vi "Main.vi"() -> ()   [LabVIEW 2020]
doc: "Cet exemple de projet Mesure continue est basé sur le modèle Gestionnaire de messages dans une file d'attente.\n\nLa boucle de gestion d'événements génère des messages en fonction des actions sur l'interface utilisateur.\n\nLa boucle de gestion de messages traite les messages générés par la boucle de gestion d'événements ou par d'autres messages. Il y a aussi des sous-VIs de boucle de gestion de messages d'acquisition et d'enregistrement, ainsi qu'une boucle de mise à jour du graphe déroulant."
uses:
  Settings/Settings.ctl
  Acquisition/Hardware Configuration.ctl
  Acquisition/Signal Type.ctl
  Logging/Logging Configuration.ctl
  controls/UI Data.ctl
  controls/UI State.ctl
  support/Message Queue/Enqueue Message (Single).vi
  support/Message Queue/Enqueue Message (Array).vi
  <vilib>/Utility/error.llb/Error Cluster From Error Code.vi
  <vilib>/ErrorRing/Error Ring.xnode
  Acquisition/Acquisition.lvlib
  Logging/Logging.lvlib
  Settings/Settings.lvlib
  support/User Event - Stop/User Event - Stop.lvlib
  support/Message Queue/Message Queue.lvlib
  Settings/Settings Dialog.vi
panel:
  in  "Panneaux":T1(tab)
  out "Chaîne":string
  in  "Moyennage sélectionneur":bool
  in  "Choix moyennage":dbl
  in  "Mode longueur d'onde":bool=TRUE
  in  "Sélectionneur de longueur d'onde":dbl=500.0 min=500.0 max=2500.0 step=1.0
  in  "Longueur d'onde":bool
  out "Données":waveform(dbl)[](graph)
  out "État":string
  in  "Quitter":bool
  in  "Arrêter":bool
  in  "Démarrer":bool
  in  "Paramètres":bool
  out "Tableau 2":dbl[](array[numeric])
  # "MAPA Tech"
  # "Automatique"
  # "Manuel"
  # "MAPA Tech"
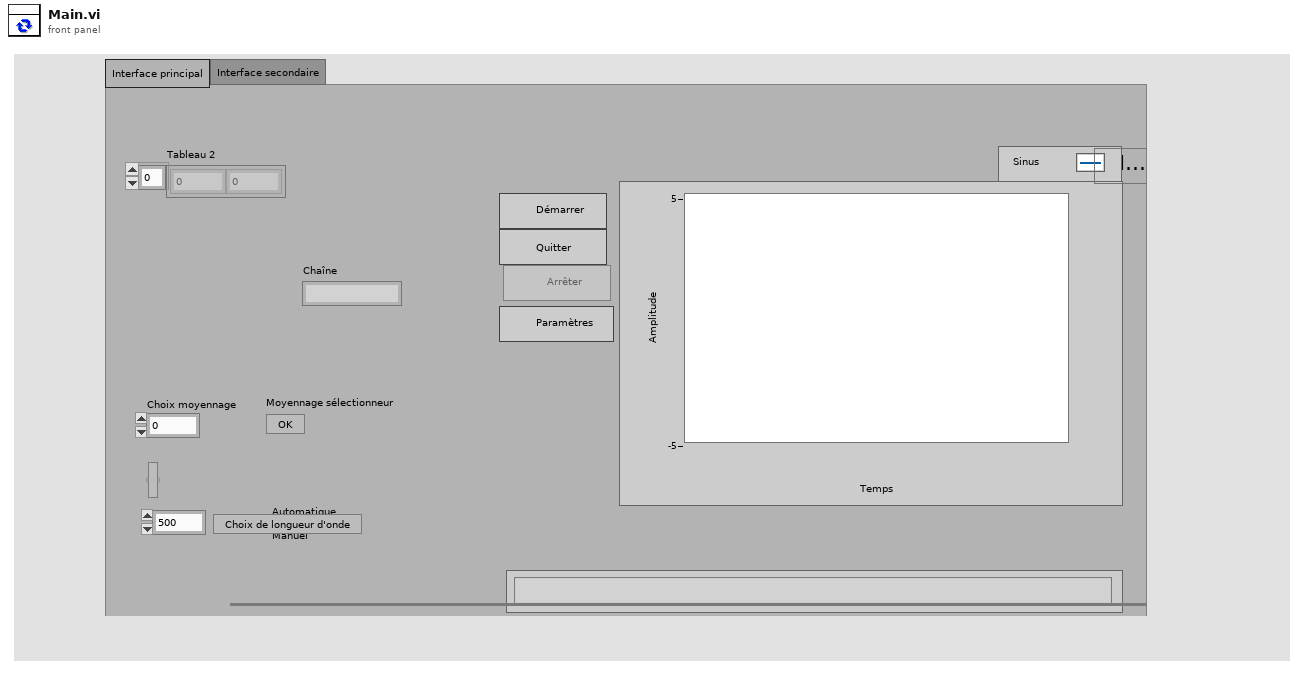
[diagram p1: front panel]
types:
  T1 = enum32{"Interface principal", "Interface secondaire"}
  T2 = typedef "UI State.ctl" = enum16{"Idle", "Acquiring and Logging", "Waiting for Exit", "Waiting for Exit (Acq Stopped)", "Waiting for Exit (Log Stopped)", "Waiting for Stop", "Waiting for Stop (Acq Stopped)", "Waiting for Stop (Log Stopped)"}
  T3 = typedef "UI Data.ctl" = cluster{"Réf. de Démarrer":refnum<vi>, "Réf. d'Arrêter":refnum<vi>, "Réf. de Paramètres":refnum<vi>, "Réf. de Quitter":refnum<vi>, "Réf. d'état":refnum<vi>, "Réf. de données":refnum<vi>, "Ref. longueur d'onde":refnum<vi>, "Ref. Choix mode longueur d'onde":refnum<vi>, "Ref. Moyennage sélectionneur":refnum<vi>}
  T4 = typedef "Settings.lvlib/Settings.ctl" = cluster{"Configuration du matériel":T5, "Configuration de l'enregistrement":T7, "Cluster test":cluster{"Numérique":dbl, "Numérique 2":dbl}, "Mode de longueur d'onde":cluster{"Choix du mode":bool}}
  T5 = typedef "Acquisition.lvlib/Hardware Configuration.ctl" = cluster{"Refnum de matériel <À remplacer>":string, "Type de signal <À remplacer>":T6}
  T6 = typedef "Acquisition.lvlib/Signal Type.ctl" = enum16{"Sine Wave", "Square with Noise", "Signal triangulaire", "Simulation DAQ"}
  T7 = typedef "Logging.lvlib/Logging Configuration.ctl" = cluster{"Chemin de base du fichier journal":path, "Référence de fichier TDMS":refnum<k34>}
  T8 = cluster{"état":bool, "code":i32, "source":string}
  T9 = typedef "Message Queue.lvlib/All Message Queues.ctl" = cluster{"IU":refnum<queue>, "Acquisition":refnum<queue>, "Enregistrement":refnum<queue>}
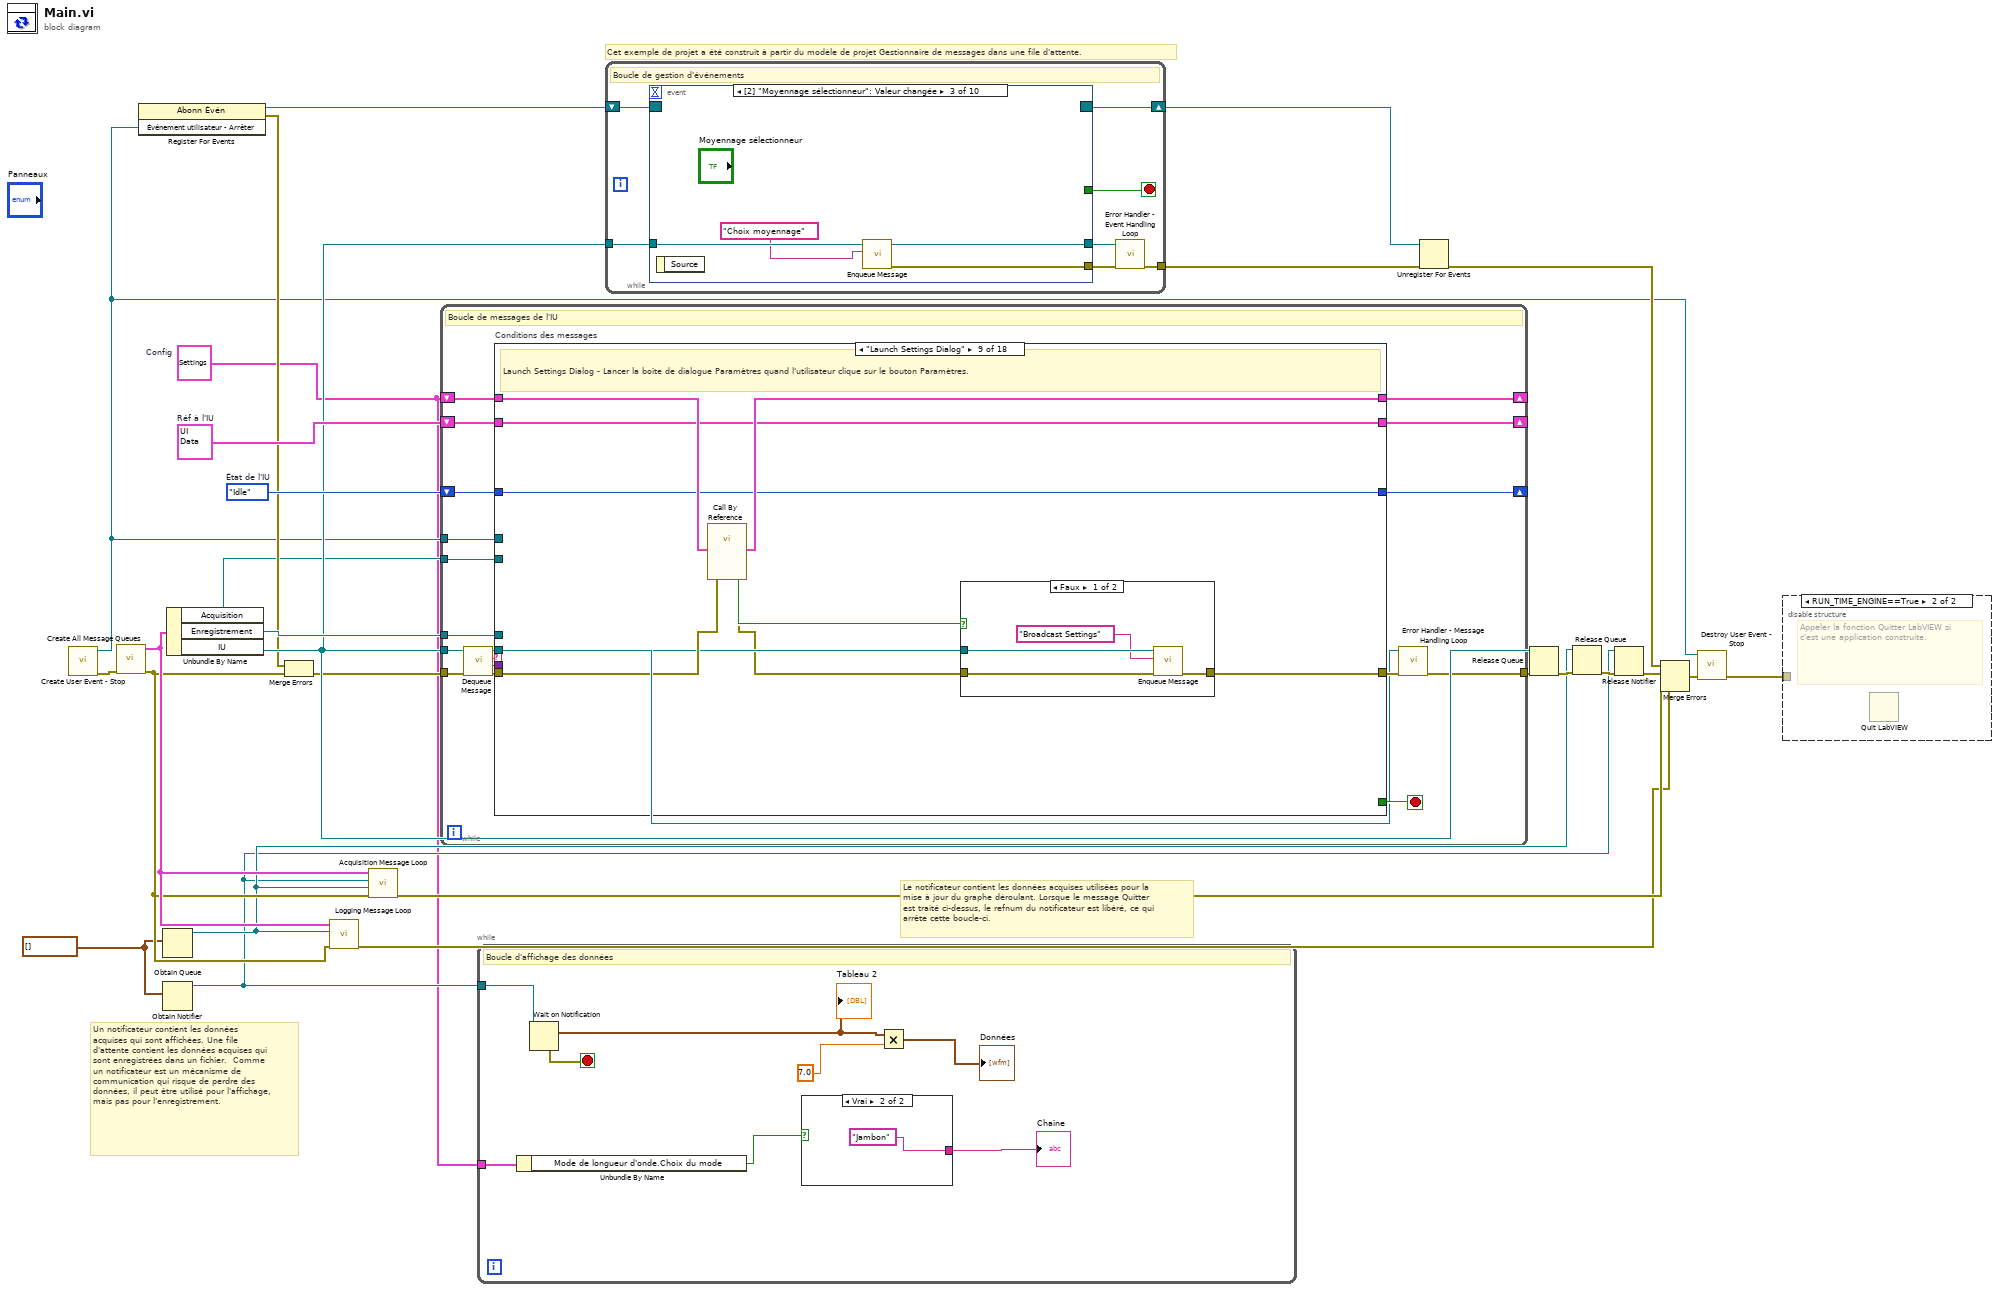
[diagram p0: block diagram]
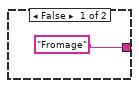
[diagram p3: hidden frame]
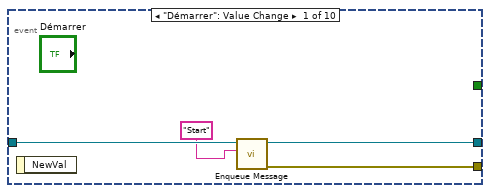
[diagram p4: hidden frame]
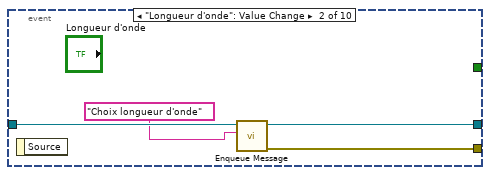
[diagram p5: hidden frame]
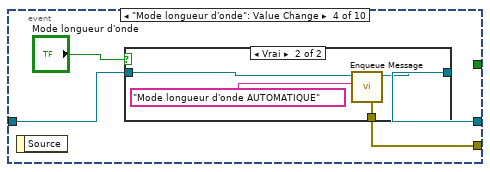
[diagram p6: hidden frame]
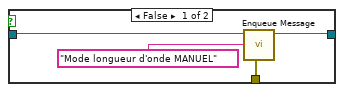
[diagram p7: hidden frame]
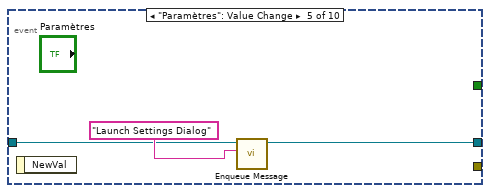
[diagram p8: hidden frame]
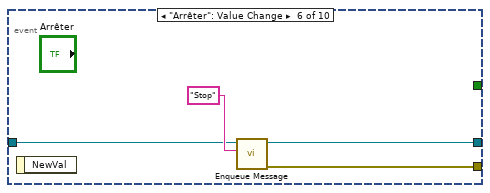
[diagram p9: hidden frame]
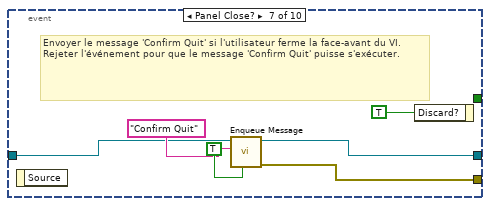
[diagram p10: hidden frame]
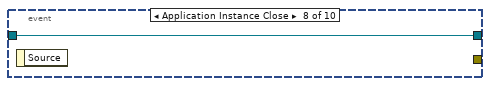
[diagram p11: hidden frame]
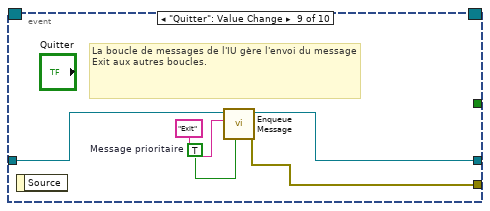
[diagram p12: hidden frame]
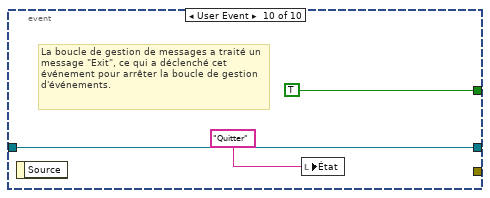
[diagram p13: hidden frame]
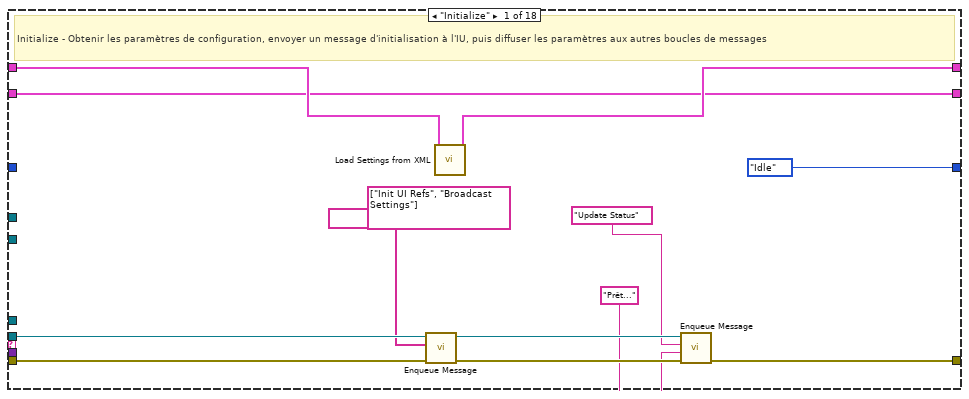
[diagram p14: hidden frame]
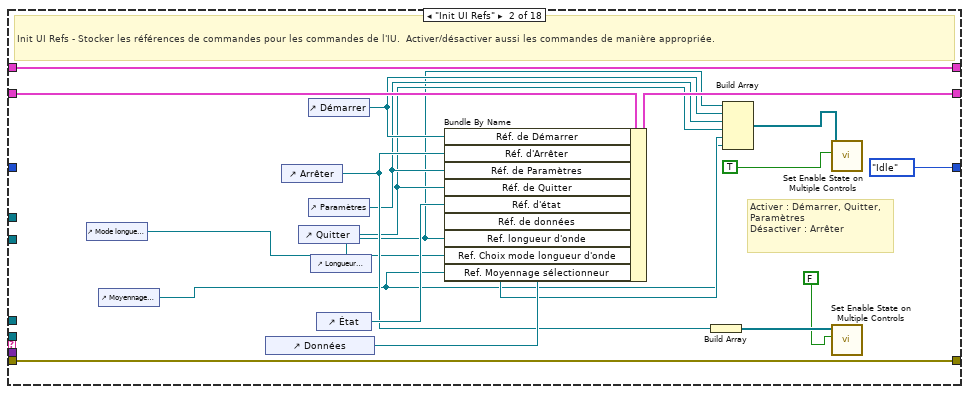
[diagram p15: hidden frame]
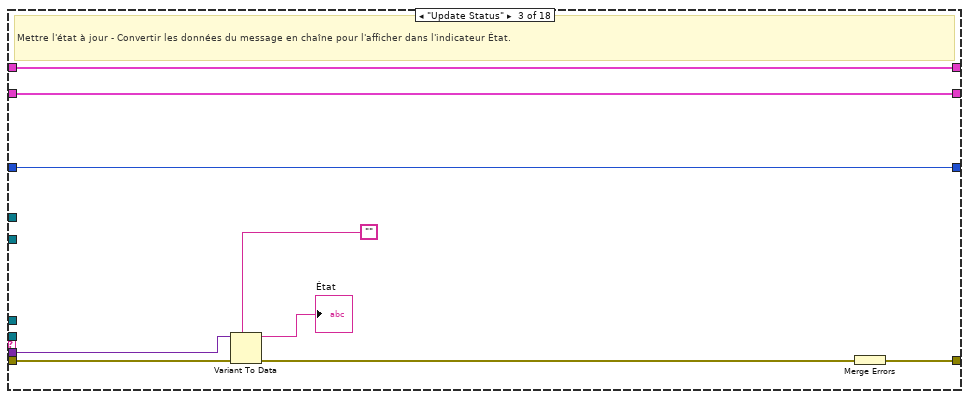
[diagram p16: hidden frame]
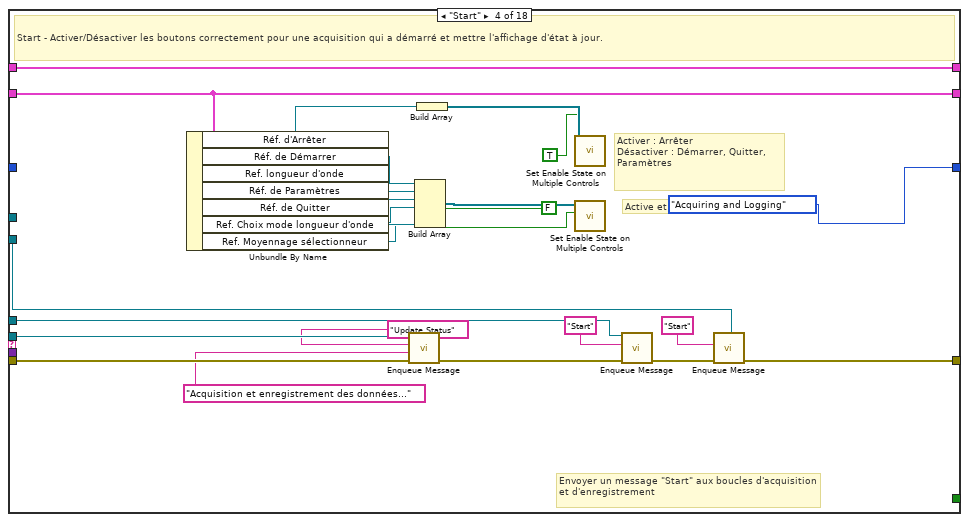
[diagram p17: hidden frame]
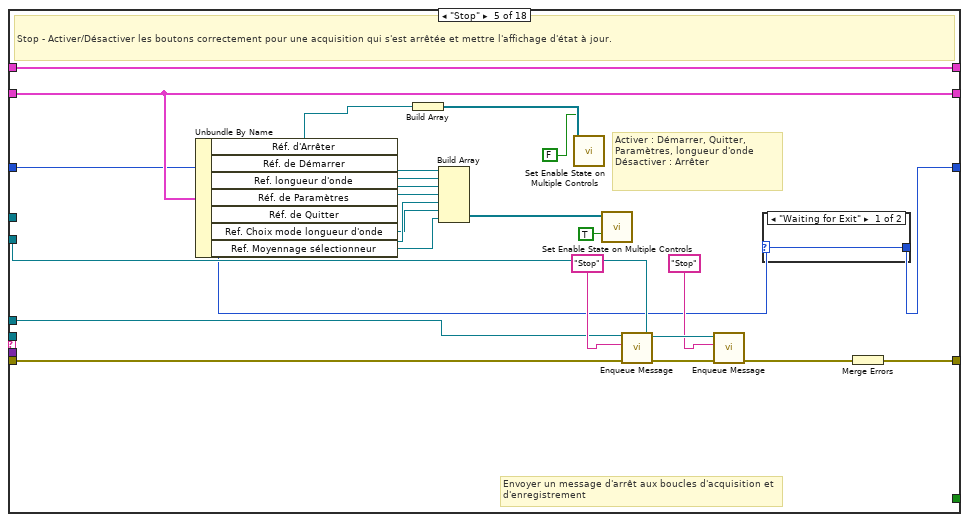
[diagram p18: hidden frame]
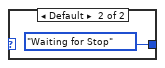
[diagram p19: hidden frame]
diagram:
  w16 = UI_State."Idle"  # État de l'IU
  w2 = waveform(dbl)[] []
  w18 = T3 {"Réf. de Démarrer"=refnum, "Réf. d'Arrêter"=refnum, "Réf. de Paramètres"=refnum, "Réf. de Quitter"=refnum, "Réf. d'état"=refnum, "Réf. de données"=refnum, "Ref. longueur d'onde"=refnum, "Ref. Choix mode longueur d'onde"=refnum, "Ref. Moyennage sélectionneur"=refnum}  # Réf à l'IU
  w1 = T4 {"Configuration du matériel"={"Refnum de matériel <À remplacer>"="", "Type de signal <À remplacer>"=enum."Simulation DAQ"}, "Configuration de l'enregistrement"={"Chemin de base du fichier journal"=path "", "Référence de fichier TDMS"=refnum}, "Cluster test"={"Numérique"=15.0, "Numérique 2"=0.0}, "Mode de longueur d'onde"={"Choix du mode"=TRUE}}  # Config
  # "Cet exemple de projet a été construit à partir du modèle de projet Gestionnaire de messages dans une file d'attente."
  # "Un notificateur contient les données acquises qui sont affichées. Une file d'attente contient les données acquises qui sont enregistrées dans un fichier.  Comme un notificateur est un mécanisme de communication qui risque de perdre des données, il peut être utilisé pour l'affichage, mais pas pour l'enregistrement."
  # "Le notificateur contient les données acquises utilisées pour la mise à jour du graphe déroulant. Lorsque le message Quitter est traité ci-dessus, le refnum du notificateur est libéré, ce qui arrête cette boucle-ci."
  n1 = call "Create User Event - Stop.vi"() -> ("error out"=w24:T8, "Événement utilisateur - Arrêter"=w3:refnum<user-event>)  [unwired: 10 in]
  n2 = call "Create All Message Queues.vi"("error in (no error)"=w24) -> ("error out"=w21:T8, "Files d'attente de messages en sortie"=w23:T9)  [unwired: 9 in]
  n3 = register-events(w3) -> (reference out=w7:refnum<event-registration>, error out=w5:errorcluster)  [unwired: 2 in]
  n4 = Obtain Queue(element data type=w2) -> (queue out=w9:refnum<queue>)  [unwired: 4 in, 2 out]
  n5 = Obtain Notifier(notification data type=w2) -> (notifier out=w8:refnum<notifier>)  [unwired: 3 in, 2 out]
  n6 = Unbundle By Name(w23) -> ("Acquisition"=w4:refnum<queue>, "Enregistrement"=w17:refnum<queue>, "IU"=w14:refnum<queue>)
  n7 = Merge Errors(w5, w21) -> (w6:errorcluster)
  n8 = call "Logging Message Loop.vi"("error in (no error)"=w21, "File d'attente de données"=w9, "Files d'attente de messages"=w23) -> ("error out"=w22:T8)  [unwired: 8 in]
  n9 = call "Acquisition Message Loop.vi"("error in (no error)"=w21, "File d'attente de données"=w9, "Notificateur de données"=w8, "Files d'attente de messages"=w23) -> ("error out"=w25:T8)  [unwired: 7 in]
  n10 = while {
    tunnel: w14 -> [w39]
    tunnel: w3 -> [w44]
    shift-right: [w38] -> _
    shift-left: w1 -> [w37]
    shift-right: [w35] -> _
    shift-left: w18 -> [w36]
    tunnel: w4 -> [w34]
    tunnel: w17 -> [w33]
    shift-right: [w28] -> _
    shift-left: w16 -> [w29]
    tunnel: w6 -> [w43]
    tunnel: [w32] -> w27
    stop <- w45 stop-if-true
    # "Boucle de messages de l'IU"
    n11 = call "Dequeue Message.vi"("error in (no error)"=w43, "File d'attente de messages"=w39) -> ("error out"=w42:T8, "Données de message"=w40:variant, "Message"=w41:string, "File d'attente de message dup."=w30:refnum<queue>)  [unwired: 6 in]
    n12 = case "Conditions des messages" shown="\"Launch Settings Dialog\"" w41 {
      selector: w41 -> [_ _ _ _ _ _ _ _ _ _ _ _ _ _ _ _ _ w347]
      tunnel: w30 -> [w49 _ _ w109 _ w137 w162 _ w204 _ w225 _ _ w288 w308 w325 w342 _]
      tunnel: w42 -> [w48 w75 w83 w108 w131 w138 w163 w192 w206 w213 w224 w253 w270 w291 w311 w328 w345 _]
      tunnel: [w53 w75 w84 w93 w132 w135 w160 w198 w199 w216 w223 w263 w269 w290 w310 w327 w344 w346] -> w31
      tunnel: [_ _ _ _ _ _ _ _ _ _ _ TRUE _ _ _ _ _ _] -> w45
      tunnel: w40 -> [_ _ w82 _ _ _ _ _ _ w217 _ w251 _ _ _ _ _ _]
      tunnel: w44 -> [_ _ _ _ _ _ _ _ _ _ _ w264 _ _ _ _ _ _]
      tunnel: [w56 w74 w78 w107 w130 w141 w166 w196 w203 w221 w228 w262 w268 w289 w309 w326 w343 w350] -> w38
      tunnel: w37 -> [w57 w74 w78 w107 w130 w141 w166 w196 w207 w221 w228 w262 w268 w289 w309 w326 w343 w350]
      tunnel: w36 -> [w50 w73 w77 w104 w129 w140 w165 w191 w201 w220 w227 w261 w267 w279 w300 w319 w336 w349]
      tunnel: [w50 w70 w77 w104 w129 w140 w165 w191 w201 w220 w227 w261 w267 w279 w300 w319 w336 w349] -> w35
      tunnel: w34 -> [_ _ _ w92 w118 _ _ w190 _ _ _ w260 _ _ _ _ _ _]
      tunnel: w33 -> [_ _ _ w95 w121 _ _ w185 _ _ _ w259 _ _ _ _ _ _]
      tunnel: w29 -> [_ _ w76 _ w115 w139 w164 w189 w200 w215 w226 _ w266 _ _ _ _ w348]
      tunnel: [UI_State."Idle" ("UI State") UI_State."Idle" ("UI State") w76 UI_State."Acquiring and Logging" ("UI State") w116 w136 w161 w189 w200 w215 w222 UI_State."Idle" ("UI State") w266 UI_State."Acquiring and Logging" ("UI State") UI_State."Acquiring and Logging" ("UI State") UI_State."Acquiring and Logging" ("UI State") UI_State."Acquiring and Logging" ("UI State") w348] -> w28
      frame "Initialize" {
        # "Initialize - Obtenir les paramètres de configuration, envoyer un message d'initialisation à l'IU, puis diffuser les paramètres aux autres boucles de messages"
        n13 = call-poly "Enqueue Message.vi"("error in (no error)"=w48, "Tableau de messages"=string[] ["Init UI Refs", "Broadcast Settings"], "File d'attente de messages"=w49) -> ("error out"=w55:T8, "File d'attente de message dup."=w54:refnum<queue>)  [unwired: 7 in]
        n14 = call "Load Settings from XML.vi"("Paramètres en entrée"=w57) -> ("Paramètres en sortie"=w56:T4)  [unwired: 9 in, 1 out]
        n15 = call-poly "Enqueue Message.vi"("error in (no error)"=w55, "Données de message"="Prêt..." ("Ready..."), "Message"="Update Status", "File d'attente de messages"=w54) -> ("error out"=w53:T8)  [unwired: 6 in, 1 out]
      }
      frame "Init UI Refs" {
        # "Activer : Démarrer, Quitter, Paramètres\nDésactiver : Arrêter"
        # "Init UI Refs - Stocker les références de commandes pour les commandes de l'IU.  Activer/désactiver aussi les commandes de manière appropriée."
        n16 = control-ref of="Mode longueur d'onde"() -> (w59:refnum<vi>)
        n17 = control-ref of="Moyennage sélectionneur"() -> (w58:refnum<vi>)
        n18 = control-ref of="Données"() -> (w71:refnum<vi>)
        n19 = control-ref of="Arrêter"() -> (w65:refnum<vi>)
        n20 = control-ref of="Quitter"() -> (w62:refnum<vi>)
        n21 = control-ref of="Démarrer"() -> (w64:refnum<vi>)
        n22 = control-ref of="Paramètres"() -> (w63:refnum<vi>)
        n23 = control-ref of="Longueur d'onde"() -> (w60:refnum<vi>)
        n24 = control-ref of="État"() -> (w72:refnum<vi>)
        n25 = Bundle By Name(cluster=w73, "Réf. de Démarrer"=w64, "Réf. d'Arrêter"=w65, "Réf. de Paramètres"=w63, "Réf. de Quitter"=w62, "Réf. d'état"=w72, "Réf. de données"=w71, "Ref. longueur d'onde"=w60, "Ref. Choix mode longueur d'onde"=w59, "Ref. Moyennage sélectionneur"=w58) -> (w70:T3)
        n26 = Build Array(w65) -> (w67:refnum<vi>[])
        n27 = Build Array(w60, w64, w63, w62, w59, w58) -> (w68:refnum<vi>[])
        n28 = call "Set Enable State on Multiple Controls.vi"("Activé ?"=TRUE ("Enable?"), "Commandes"=w68) -> ()  [unwired: 10 in]
        n29 = call "Set Enable State on Multiple Controls.vi"("Activé ?"=FALSE ("Enable?"), "Commandes"=w67) -> ()  [unwired: 10 in]
      }
      frame "Update Status" {
        # "Mettre l'état à jour - Convertir les données du message en chaîne pour l'afficher dans l'indicateur État."
        n30 = Variant To Data(error in=w83, type="" ("Empty String Constant"), Variant=w82) -> (data=→"État":string, error out=w80:errorcluster)
        n31 = Merge Errors(w80) -> (w84:errorcluster)
      }
      frame "Start" {
        # "Active et désactive les boutons!"
        # "Envoyer un message \"Start\" aux boucles d'acquisition et d'enregistrement"
        # "Activer : Arrêter\nDésactiver : Démarrer, Quitter, Paramètres"
        # "Start - Activer/Désactiver les boutons correctement pour une acquisition qui a démarré et mettre l'affichage d'état à jour."
        n32 = Unbundle By Name(w104) -> ("Réf. d'Arrêter"=w99:refnum<vi>, "Réf. de Démarrer"=w98:refnum<vi>, "Ref. longueur d'onde"=w89:refnum<vi>, "Réf. de Paramètres"=w88:refnum<vi>, "Réf. de Quitter"=w87:refnum<vi>, "Ref. Choix mode longueur d'onde"=w86:refnum<vi>, "Ref. Moyennage sélectionneur"=w85:refnum<vi>)
        n33 = call-poly "Enqueue Message.vi"("error in (no error)"=w108, "Données de message"="Acquisition et enregistrement des données..." ("Acquiring and Logging..."), "Message"="Update Status", "File d'attente de messages"=w109) -> ("error out"=w97:T8)  [unwired: 6 in, 1 out]
        n34 = Build Array(w98, w89, w88, w87, w86, w85) -> (w102:refnum<vi>[])
        n35 = Build Array(w99) -> (w101:refnum<vi>[])
        n36 = call "Set Enable State on Multiple Controls.vi"("Activé ?"=TRUE ("Enable?"), "Commandes"=w101) -> ()  [unwired: 10 in]
        n37 = call "Set Enable State on Multiple Controls.vi"("Activé ?"=FALSE ("Enable?"), "Commandes"=w102) -> ()  [unwired: 10 in]
        n38 = call-poly "Enqueue Message.vi"("error in (no error)"=w97, "Message"="Start", "File d'attente de messages"=w95) -> ("error out"=w94:T8)  [unwired: 7 in, 1 out]
        n39 = call-poly "Enqueue Message.vi"("error in (no error)"=w94, "Message"="Start", "File d'attente de messages"=w92) -> ("error out"=w93:T8)  [unwired: 7 in, 1 out]
      }
      frame "Stop" {
        # "Envoyer un message d'arrêt aux boucles d'acquisition et d'enregistrement"
        # "Activer : Démarrer, Quitter, Paramètres, longueur d'onde\nDésactiver : Arrêter"
        # "Stop - Activer/Désactiver les boutons correctement pour une acquisition qui s'est arrêtée et mettre l'affichage d'état à jour."
        n40 = Unbundle By Name(w129) -> ("Réf. d'Arrêter"=w124:refnum<vi>, "Réf. de Démarrer"=w123:refnum<vi>, "Ref. longueur d'onde"=w114:refnum<vi>, "Réf. de Paramètres"=w113:refnum<vi>, "Réf. de Quitter"=w112:refnum<vi>, "Ref. Choix mode longueur d'onde"=w111:refnum<vi>, "Ref. Moyennage sélectionneur"=w110:refnum<vi>)
        n41 = Build Array(w124) -> (w126:refnum<vi>[])
        n42 = Build Array(w114, w123, w114, w113, w112, w111, w110) -> (w127:refnum<vi>[])
        n43 = call "Set Enable State on Multiple Controls.vi"("Activé ?"=FALSE ("Enable?"), "Commandes"=w126) -> ()  [unwired: 10 in]
        n44 = call "Set Enable State on Multiple Controls.vi"("Activé ?"=TRUE ("Enable?"), "Commandes"=w127) -> ()  [unwired: 10 in]
        n45 = call-poly "Enqueue Message.vi"("error in (no error)"=w131, "Message"="Stop", "File d'attente de messages"=w121) -> ("error out"=w120:T8)  [unwired: 7 in, 1 out]
        n46 = call-poly "Enqueue Message.vi"("error in (no error)"=w120, "Message"="Stop", "File d'attente de messages"=w118) -> ("error out"=w119:T8)  [unwired: 7 in, 1 out]
        n47 = case shown="\"Waiting for Exit\"" w115 {
          selector: w115 -> [w133 _]
          tunnel: [w133 UI_State."Waiting for Stop" ("UI State")] -> w116
          frame "Waiting for Exit" {
          }
          frame Default {
          }
        }
        n48 = Merge Errors(w119) -> (w132:errorcluster)
      }
      frame "Acquisition Stopped" {
        # "Logique déterminant quelle action entreprendre quand l'acquisition s'est arrêtée."
        n49 = case shown="Par défaut" w139 {
          selector: w139 -> [w143 _ _ _ _]
          tunnel: w138 -> [w142 w145 w147 w153 w159]
          tunnel: w137 -> [_ _ _ w151 w156]
          tunnel: [w143 UI_State."Waiting for Exit (Acq Stopped)" ("UI State") UI_State."Waiting for Stop (Acq Stopped)" ("UI State") UI_State."Idle" ("UI State") UI_State."Idle" ("UI State")] -> w136
          tunnel: [w142 w145 w147 w152 w157] -> w135
          frame Default {
          }
          frame "Waiting for Exit", "Waiting for Exit (Acq Stopped)" {
          }
          frame "Waiting for Stop", "Waiting for Stop (Acq Stopped)" {
          }
          frame "Waiting for Exit (Log Stopped)" {
            # "Si nous attendons pour quitter et que l'enregistrement s'est déjà arrêté, le message \"Acquisition Stopped\" indique qu'il est temps de quitter."
            n50 = call-poly "Enqueue Message.vi"("Message prioritaire ? (F)"=TRUE ("Priority Message? (F)"), "error in (no error)"=w153, "Message"="Exit", "File d'attente de messages"=w151) -> ("error out"=w152:T8)  [unwired: 6 in, 1 out]
          }
          frame "Waiting for Stop (Log Stopped)" {
            # "Si nous attendons pour arrêter et que l'enregistrement s'est déjà arrêté, le message \"Acquisition Stopped\" indique qu'il est temps d'arrêter."
            n51 = call-poly "Enqueue Message.vi"("error in (no error)"=w159, "Données de message"="Prêt..." ("Ready..."), "Message"="Update Status", "File d'attente de messages"=w156) -> ("error out"=w157:T8)  [unwired: 6 in, 1 out]
          }
        }
      }
      frame "Logging Stopped" {
        # "Logique déterminant quelle action entreprendre quand l'enregistrement s'est arrêté."
        n52 = case shown="\"Waiting for Stop (Acq Stopped)\"" w164 {
          selector: w164 -> [w168 _ _ _ _]
          tunnel: w163 -> [w167 w170 w172 w178 w181]
          tunnel: w162 -> [_ _ _ w176 w180]
          tunnel: [w168 UI_State."Waiting for Exit (Log Stopped)" ("UI State") UI_State."Waiting for Stop (Log Stopped)" ("UI State") UI_State."Idle" ("UI State") UI_State."Idle" ("UI State")] -> w161
          tunnel: [w167 w170 w172 w177 w179] -> w160
          frame Default {
          }
          frame "Waiting for Exit", "Waiting for Exit (Log Stopped)" {
          }
          frame "Waiting for Stop", "Waiting for Stop (Log Stopped)" {
          }
          frame "Waiting for Exit (Acq Stopped)" {
            # "Si nous attendons pour quitter et que l'acquisition s'est déjà arrêtée, le message \"Logging Stopped\" indique qu'il est temps de quitter."
            n53 = call-poly "Enqueue Message.vi"("Message prioritaire ? (F)"=TRUE ("Priority Message? (F)"), "error in (no error)"=w178, "Message"="Exit", "File d'attente de messages"=w176) -> ("error out"=w177:T8)  [unwired: 6 in, 1 out]
          }
          frame "Waiting for Stop (Acq Stopped)" {
            # "Si nous attendons pour arrêter et que l'acquisition s'est déjà arrêtée, le message \"Logging Stopped\" indique qu'il est temps d'arrêter."
            n54 = call-poly "Enqueue Message.vi"("error in (no error)"=w181, "Données de message"="Prêt..." ("Ready..."), "Message"="Update Status", "File d'attente de messages"=w180) -> ("error out"=w179:T8)  [unwired: 6 in, 1 out]
          }
        }
      }
      frame "Broadcast settings" {
        w186 = "Update Settings" ("Message")
        # "Broadcast settings - Envoyer le message 'Update Settings' aux boucles de messages d'enregistrement et d'acquisition."
        n55 = Unbundle By Name(w196) -> ("Configuration du matériel"=w195:T5, "Configuration de l'enregistrement"=w194:T7, "Mode de longueur d'onde"=w188:cluster{"Choix du mode":bool})
        n56 = call-poly "Enqueue Message.vi"("Données de message"=w188, "Message"=w186, "File d'attente de messages"=w185) -> ("error out"=w187:T8)  [unwired: 7 in, 1 out]
        n57 = call-poly "Enqueue Message.vi"("Données de message"=w195, "Message"=w186, "File d'attente de messages"=w190) -> ("error out"=w197:T8)  [unwired: 7 in, 1 out]
        n58 = call-poly "Enqueue Message.vi"("error in (no error)"=w197, "Données de message"=w194, "Message"=w186, "File d'attente de messages"=w185) -> ("error out"=w193:T8)  [unwired: 6 in, 1 out]
        n59 = Merge Errors(w187, w193, w192) -> (w198:errorcluster)
      }
      frame "Launch Settings Dialog" {
        # "Launch Settings Dialog - Lancer la boîte de dialogue Paramètres quand l'utilisateur clique sur le bouton Paramètres."
        n60 = call-by-ref "?"("error in (no error)"=w206, "Paramètres en entrée"=w207) -> ("error out"=w202:T8, "Annulation ?"=w205:bool, "Paramètres en sortie"=w203:T4)  [unwired: 8 in, 3 out]
        n61 = case shown="Faux" w205 {
          tunnel: w204 -> [w211 _]
          tunnel: w202 -> [w210 w212]
          tunnel: [w209 w212] -> w199
          frame False {
            n62 = call-poly "Enqueue Message.vi"("error in (no error)"=w210, "Message"="Broadcast Settings", "File d'attente de messages"=w211) -> ("error out"=w209:T8)  [unwired: 7 in, 1 out]
          }
          frame True {
          }
        }
      }
      frame "Error" {
        # "Error - Afficher une boîte de dialogue d'erreur. Ce message est envoyé par les VIs \"Error Handler\" à la fin de l'exécution de chaque boucle de cette application."
        n63 = Variant To Data(error in=w213, type=errorcluster {"status"=FALSE, "code"=0, "source"=""} ("error constant"), Variant=w217) -> (data=w214:errorcluster, error out=w218:errorcluster)
        n64 = call <vilib>:"Simple Error Handler.vi"("error in (no error)"=w214) -> ()  [unwired: 4 in, 5 out]
        n65 = Merge Errors(w218) -> (w216:errorcluster)
      }
      frame "Confirm Quit" {
        # "Confirm Quit - Message qui confirme si l'utilisateur voulait vraiment quitter l'application."
        n66 = case shown="\"Acquiring and Logging\"" w226 {
          tunnel: w225 -> [w234 w238]
          tunnel: w224 -> [w233 w237]
          tunnel: [w232 w236] -> w223
          tunnel: [UI_State."Idle" ("UI State") w235] -> w222
          frame Default {
            # "Si 'Confirm Quit' survient alors que le système est inactif, le message de confirmation est inutile."
            n67 = call-poly "Enqueue Message.vi"("Message prioritaire ? (F)"=TRUE ("Priority Message? (F)"), "error in (no error)"=w233, "Message"="Exit", "File d'attente de messages"=w234) -> ("error out"=w232:T8)  [unwired: 6 in, 1 out]
          }
          frame "Acquiring and Logging" {
            n68 = Two Button Dialog(message="Voulez-vous vraiment quitter en cours d'acquisition ?" ("Confirm Quit Message"), 1:"Non" ("No"), 2:"Oui" ("Yes")) -> (T button?=w239:bool)
            n69 = case shown="Vrai" w239 {
              tunnel: w238 -> [_ w248]
              tunnel: w237 -> [w244 w249]
              tunnel: [w244 w247] -> w236
              tunnel: [UI_State."Acquiring and Logging" ("UI State") UI_State."Waiting for Exit" ("UI State")] -> w235
              frame False {
                # "L'utilisateur ne voulait pas quitter."
              }
              frame True {
                n70 = call-poly "Enqueue Message.vi"("error in (no error)"=w249, "Message"="Stop", "File d'attente de messages"=w248) -> ("error out"=w247:T8)  [unwired: 7 in, 1 out]
              }
            }
          }
        }
      }
      frame "Exit" {
        w255 = TRUE ("Priority Message? (F)")
        w256 = "Exit" ("Message")
        # "Afficher une boîte de dialogue d'erreur si 'Exit' a été appelé suite à une erreur."
        # "Arrêter le VI"
        # "Exit - Envoyer des messages Exit aux boucles d'acquisition et d'enregistrerment, et déclencher l'événement utilisateur pour arrêter la boucle de gestion d'événements."
        n71 = Variant To Data(type=errorcluster {"status"=FALSE, "code"=0, "source"=""} ("error constant"), Variant=w251) -> (data=w250:errorcluster)  [unwired: 1 in, 1 out]
        n72 = call <vilib>:"Simple Error Handler.vi"("error in (no error)"=w250) -> ()  [unwired: 4 in, 5 out]
        n73 = call-poly "Enqueue Message.vi"("Message prioritaire ? (F)"=w255, "error in (no error)"=w253, "Message"=w256, "File d'attente de messages"=w260) -> ("error out"=w257:T8)  [unwired: 6 in, 1 out]
        n74 = call-poly "Enqueue Message.vi"("Message prioritaire ? (F)"=w255, "error in (no error)"=w257, "Message"=w256, "File d'attente de messages"=w259) -> ("error out"=w254:T8)  [unwired: 6 in, 1 out]
        n75 = call "Fire User Event - Stop.vi"("error in (no error)"=w254, "Événement utilisateur - Arrêt"=w264) -> ("error out"=w263:T8)  [unwired: 9 in]
      }
      frame "---Copy This Frame---" {
        # "Dupliquez cette étape pour créer de nouveaux messages.  Changez ce commentaire dans l'étape dupliquée pour décrire ce message."
        n76 = Merge Errors(w270) -> (w269:errorcluster)
      }
      frame "Choix longueur d'onde" {
        # "Activer : \nDésactiver :"
        # "Affiche la longueur d'onde en live.\nComment je fais pour limiter le range\ncomment je fais pour afficher pas en live\ngestion d'erreur?"
        # "Dupliquez cette étape pour créer de nouveaux messages.  Changez ce commentaire dans l'étape dupliquée pour décrire ce message."
        n77 = Unbundle By Name(w279) -> ("Ref. longueur d'onde"=w276:refnum<vi>, "Réf. d'Arrêter"=w274:refnum<vi>, "Réf. de Démarrer"=w273:refnum<vi>, "Réf. de Quitter"=w277:refnum<vi>, "Réf. de Paramètres"=w275:refnum<vi>)
        n78 = Build Array(w273, w277, w276, w275) -> (w281:refnum<vi>[])
        n79 = Build Array(w274) -> (w272:refnum<vi>[])
        n80 = call "Set Enable State on Multiple Controls.vi"("Activé ?"=TRUE ("Enable?"), "Commandes"=w281) -> ()  [unwired: 10 in]
        n81 = Number To Decimal String(number="Sélectionneur de longueur d'onde") -> (decimal integer string=w285:string)  [unwired: 1 in]
        n82 = Concatenate Strings ("Concaténer des chaînes")("La longueur d'onde sélectionné est de ", w285, " nm.") -> (w282:string)
        n83 = call "Set Enable State on Multiple Controls.vi"("Activé ?"=FALSE ("Enable?"), "Commandes"=w272) -> ()  [unwired: 10 in]
        n84 = call-poly "Enqueue Message.vi"("Données de message"=w282, "Message"="Update Status", "File d'attente de messages"=w288) -> ()  [unwired: 7 in, 2 out]
        n85 = Merge Errors(w291) -> (w290:errorcluster)
      }
      frame "Choix moyennage" {
        # "Activer : \nDésactiver :"
        # "Affiche la longueur d'onde en live.\nComment je fais pour limiter le range\ncomment je fais pour afficher pas en live\ngestion d'erreur?"
        # "Dupliquez cette étape pour créer de nouveaux messages.  Changez ce commentaire dans l'étape dupliquée pour décrire ce message."
        n86 = Unbundle By Name(w300) -> ("Réf. d'Arrêter"=w294:refnum<vi>, "Réf. de Démarrer"=w293:refnum<vi>, "Réf. de Quitter"=w298:refnum<vi>, "Réf. de Paramètres"=w292:refnum<vi>)
        n87 = Build Array(w293, w298, w292) -> (w302:refnum<vi>[])
        n88 = Build Array(w294) -> (w296:refnum<vi>[])
        n89 = call "Set Enable State on Multiple Controls.vi"("Activé ?"=TRUE ("Enable?"), "Commandes"=w302) -> ()  [unwired: 10 in]
        n90 = Number To Decimal String(number="Choix moyennage") -> (decimal integer string=w306:string)  [unwired: 1 in]
        n91 = call "Set Enable State on Multiple Controls.vi"("Activé ?"=FALSE ("Enable?"), "Commandes"=w296) -> ()  [unwired: 10 in]
        n92 = Concatenate Strings ("Concaténer des chaînes")("Le moyennage sélectionné est de ", w306, " Hz.") -> (w303:string)
        n93 = call-poly "Enqueue Message.vi"("Données de message"=w303, "Message"="Update Status", "File d'attente de messages"=w308) -> ()  [unwired: 7 in, 2 out]
        n94 = Merge Errors(w311) -> (w310:errorcluster)
      }
      frame "Mode longueur d'onde AUTOMATIQUE" {
        # "Activer : \nDésactiver :"
        # "Dupliquez cette étape pour créer de nouveaux messages.  Changez ce commentaire dans l'étape dupliquée pour décrire ce message."
        n95 = Unbundle By Name(w319) -> ("Ref. longueur d'onde"=w316:refnum<vi>, "Réf. d'Arrêter"=w314:refnum<vi>, "Réf. de Démarrer"=w313:refnum<vi>, "Réf. de Quitter"=w317:refnum<vi>, "Réf. de Paramètres"=w312:refnum<vi>)
        n96 = Build Array(w313, w317, w312) -> (w321:refnum<vi>[])
        n97 = Build Array(w314, w316) -> (w322:refnum<vi>[])
        n98 = call "Set Enable State on Multiple Controls.vi"("Activé ?"=TRUE ("Enable?"), "Commandes"=w321) -> ()  [unwired: 10 in]
        n99 = call "Set Enable State on Multiple Controls.vi"("Activé ?"=FALSE ("Enable?"), "Commandes"=w322) -> ()  [unwired: 10 in]
        n100 = call-poly "Enqueue Message.vi"("Données de message"="Le mode sélectionné pour la longueur d'onde est automatique.", "Message"="Update Status", "File d'attente de messages"=w325) -> ()  [unwired: 7 in, 2 out]
        n101 = Merge Errors(w328) -> (w327:errorcluster)
      }
      frame "Mode longueur d'onde MANUEL" {
        # "Activer : \nDésactiver :"
        # "Affiche la longueur d'onde en live.\nComment je fais pour limiter le range\ncomment je fais pour afficher pas en live\ngestion d'erreur?"
        # "Dupliquez cette étape pour créer de nouveaux messages.  Changez ce commentaire dans l'étape dupliquée pour décrire ce message."
        n102 = Unbundle By Name(w336) -> ("Ref. longueur d'onde"=w332:refnum<vi>, "Réf. d'Arrêter"=w331:refnum<vi>, "Réf. de Démarrer"=w330:refnum<vi>, "Réf. de Quitter"=w334:refnum<vi>, "Réf. de Paramètres"=w329:refnum<vi>)
        n103 = Build Array(w329, w330, w334, w332) -> (w338:refnum<vi>[])
        n104 = Build Array(w331) -> (w339:refnum<vi>[])
        n105 = call "Set Enable State on Multiple Controls.vi"("Activé ?"=TRUE ("Enable?"), "Commandes"=w338) -> ()  [unwired: 10 in]
        n106 = call "Set Enable State on Multiple Controls.vi"("Activé ?"=FALSE ("Enable?"), "Commandes"=w339) -> ()  [unwired: 10 in]
        n107 = call-poly "Enqueue Message.vi"("Données de message"="Le mode sélectionné pour la longueur d'onde est manuel.", "Message"="Update Status", "File d'attente de messages"=w342) -> ()  [unwired: 7 in, 2 out]
        n108 = Merge Errors(w345) -> (w344:errorcluster)
      }
      frame Default {
        # "La condition 'Par défaut' ne s'exécute que s'il y a un message qui n'est défini dans aucune des autres conditions.  Renvoyer une erreur de programmation."
        n109 = xnode ("Error Ring")("paramètre 0"=w347) -> ("sortie d'erreur"=w346:errorcluster)
      }
    }
    n110 = call "Error Handler - Message Handling Loop.vi"("error in (no error)"=w31, "File d'attente de messages"=w30) -> ("erreur en entrée dup."=w32:T8)  [unwired: 8 in, 1 out]
  }
  n111 = while "Data Display Loop" {
    tunnel: w8 -> [w364]
    tunnel: w1 -> [w363]
    stop <- w365 stop-if-true
    # "Boucle d'affichage des données"
    n112 = Unbundle By Name(w363) -> ("Mode de longueur d'onde.Choix du mode"=w362:bool)
    n113 = Wait on Notification(notifier=w364) -> (notification=w360:waveform(dbl)[], error out=w365:errorcluster)  [unwired: 3 in, 2 out]
    "Tableau 2" <- w360
    n114 = case shown="Vrai" w362 {
      tunnel: ["Fromage" "Jambon"] -> w361
      frame False {
      }
      frame True {
      }
    }
    "Chaîne" <- w361
    n115 = Multiply(x=w360, y=7.0) -> (x*y=→"Données":waveform(dbl)[])
  }
  n116 = while {
    tunnel: w14 -> [w373]
    tunnel: [w370] -> w26
    shift-right: [w372] -> w19
    shift-left: w7 -> [w374]
    stop <- w371 stop-if-true
    # "Boucle de gestion d'événements"
    n117 = event shown="[2] \"Moyennage sélectionneur\": Valeur changée" {
      selector: w374 -> [_ _ _ _ _ _ _ _ _ _]
      dyn-events: [_ _ _ _ _ _ _ _ _ _] -> w372
      timeout: _ -> [_ _ _ _ _ _ _ _ _ _]
      tunnel: [_ _ _ _ _ _ _ _ _ TRUE ("Discard?")] -> w371
      tunnel: w373 -> [w378 w382 w386 w389 w400 w404 w409 w412 w414 w418]
      tunnel: [w376 w380 w384 w388 _ w403 w407 _ w417 _] -> w369
      tunnel: [w375 w379 w383 w387 w399 w402 w408 w412 w413 w418] -> w368
      event "Démarrer": Value Change {
        n118 = event-data() -> ()  [unwired: 1 in, 1 out]
        n119 = call-poly "Enqueue Message.vi"("Message"="Start", "File d'attente de messages"=w378) -> ("error out"=w376:T8, "File d'attente de message dup."=w375:refnum<queue>)  [unwired: 8 in]
      }
      event "Longueur d'onde": Value Change {
        n120 = event-data() -> ()  [unwired: 1 in, 1 out]
        n121 = call-poly "Enqueue Message.vi"("Message"="Choix longueur d'onde", "File d'attente de messages"=w382) -> ("error out"=w380:T8, "File d'attente de message dup."=w379:refnum<queue>)  [unwired: 8 in]
      }
      event "Moyennage sélectionneur": Value Change {
        n122 = event-data() -> ()  [unwired: 1 in, 1 out]
        n123 = call-poly "Enqueue Message.vi"("Message"="Choix moyennage", "File d'attente de messages"=w386) -> ("error out"=w384:T8, "File d'attente de message dup."=w383:refnum<queue>)  [unwired: 8 in]
      }
      event "Mode longueur d'onde": Value Change {
        n124 = event-data() -> ()  [unwired: 1 in, 1 out]
        n125 = case shown="Vrai" "Mode longueur d'onde" {
          tunnel: w389 -> [w393 w398]
          tunnel: [w391 w397] -> w388
          tunnel: [w392 w396] -> w387
          frame False {
            n126 = call-poly "Enqueue Message.vi"("Message"="Mode longueur d'onde MANUEL", "File d'attente de messages"=w393) -> ("error out"=w391:T8, "File d'attente de message dup."=w392:refnum<queue>)  [unwired: 8 in]
          }
          frame True {
            n127 = call-poly "Enqueue Message.vi"("Message"="Mode longueur d'onde AUTOMATIQUE", "File d'attente de messages"=w398) -> ("error out"=w397:T8, "File d'attente de message dup."=w396:refnum<queue>)  [unwired: 8 in]
          }
        }
      }
      event "Paramètres": Value Change {
        n128 = event-data() -> ()  [unwired: 1 in, 1 out]
        n129 = call-poly "Enqueue Message.vi"("Message"="Launch Settings Dialog", "File d'attente de messages"=w400) -> ("File d'attente de message dup."=w399:refnum<queue>)  [unwired: 8 in, 1 out]
      }
      event "Arrêter": Value Change {
        n130 = event-data() -> ()  [unwired: 1 in, 1 out]
        n131 = call-poly "Enqueue Message.vi"("Message"="Stop", "File d'attente de messages"=w404) -> ("error out"=w403:T8, "File d'attente de message dup."=w402:refnum<queue>)  [unwired: 8 in]
      }
      event Panel Close? {
        # "Envoyer le message 'Confirm Quit' si l'utilisateur ferme la face-avant du VI. Rejeter l'événement pour que le message 'Confirm Quit' puisse s'exécuter."
        n132 = event-data() -> ()  [unwired: 1 in, 1 out]
        n133 = call-poly "Enqueue Message.vi"("Message prioritaire ? (F)"=TRUE ("Priority Message? (F)"), "Message"="Confirm Quit", "File d'attente de messages"=w409) -> ("error out"=w407:T8, "File d'attente de message dup."=w408:refnum<queue>)  [unwired: 7 in]
        n134 = event-data ("Event Filter Node")("Discard?"=TRUE) -> ()  [unwired: 1 in, 1 out]
      }
      event Application Instance Close {
        n135 = event-data() -> ()  [unwired: 1 in, 1 out]
      }
      event "Quitter": Value Change {
        w415 = TRUE  # Message prioritaire
        # "La boucle de messages de l'IU gère l'envoi du message Exit aux autres boucles."
        n136 = event-data() -> ()  [unwired: 1 in, 1 out]
        n137 = call-poly "Enqueue Message.vi"("Message prioritaire ? (F)"=w415, "Message"="Exit", "File d'attente de messages"=w414) -> ("error out"=w417:T8, "File d'attente de message dup."=w413:refnum<queue>)  [unwired: 7 in]
      }
      event User Event {
        # "La boucle de gestion de messages a traité un message \"Exit\", ce qui a déclenché cet événement pour arrêter la boucle de gestion d'événements."
        n138 = event-data() -> ()  [unwired: 1 in, 1 out]
        n139 = local write "État"("Quitter" ("Exit String")) -> ()
      }
    }
    n140 = call "Error Handler - Event Handling Loop.vi"("error in (no error)"=w369, "File d'attente de messages"=w368) -> ("erreur en entrée dup."=w370:T8)  [unwired: 8 in, 1 out]
  }
  n141 = Unregister For Events(event registration refnum=w19, error in=w26) -> (error out=w20:errorcluster)
  n142 = Release Queue(queue=w14, error in (no error)=w27) -> (error out=w12:errorcluster)  [unwired: 1 in, 2 out]
  n143 = Release Queue(queue=w9, error in (no error)=w12) -> (error out=w11:errorcluster)  [unwired: 1 in, 2 out]
  n144 = Release Notifier(notifier=w8, error in (no error)=w11) -> (error out=w10:errorcluster)  [unwired: 1 in, 2 out]
  n145 = Merge Errors(w20, w10, w25, w22) -> (w15:errorcluster)
  n146 = call "Destroy User Event - Stop.vi"("error in (no error)"=w15, "Événement utilisateur - Arrêt"=w3) -> ("error out"=w13:T8)  [unwired: 9 in]
  n147 = disable-structure "Conditional Disable Structure" shown="RUN_TIME_ENGINE==True" {
    disable-tunnel: w13 -> [_ _]
    frame condition #0 (active) {
    }
    frame condition #1 {
      # "Appeler la fonction Quitter LabVIEW si c'est une application construite."
      n148 = Quit LabVIEW() -> ()  [unwired: 1 in]
    }
  }
